vi "FlatToRichw4lvgrpc_Msg_ToServer_2.vi"(5 "OutputClusterType":T1, 11 "InputCluster":T2) -> (3 "OutputCluster":T1)   [LabVIEW 2019, in "Generated_server.lvlib"]
uses:
  Generated_server.lvlib
  w4lvgrpc_Msg_ToServer_2.ctl
  w4lvgrpc_Msg_ToServer_2_Flat.ctl
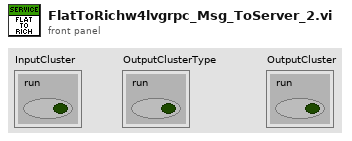
[diagram p1: front panel]
types:
  T1 = typedef "Generated_server.lvlib/w4lvgrpc_Msg_ToServer_2.ctl" = cluster{"run":bool}
  T2 = typedef "Generated_server.lvlib/w4lvgrpc_Msg_ToServer_2_Flat.ctl" = cluster{"run":bool}
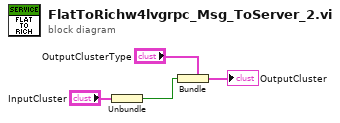
[diagram p0: block diagram]
diagram:
  n1 = Unbundle "Unbundle"("InputCluster") -> ("run"=w1:bool)
  n2 = Bundle "Bundle"(cluster="OutputClusterType", "run"=w1) -> (→"OutputCluster":T1)
